vi "Finish.vi"(8 "error in (no error)":errorcluster, 11 "Turret in":refnum<class "Turret.lvclass">) -> (0 "error out":errorcluster, 3 "Turret out":refnum<class "Turret.lvclass">)   [LabVIEW 2019, in "Turret.lvlib" / "Turret.lvclass"]
uses:
  Turret.lvclass
  Turret.lvclass/Turret.ctl
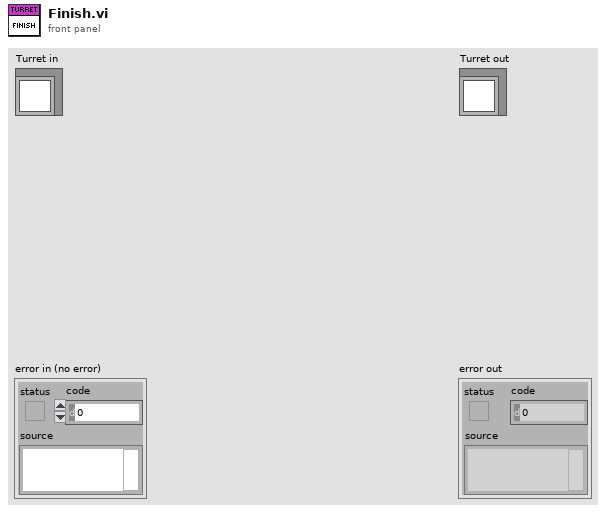
[diagram p1: front panel]
types:
  T1 = typedef "WPI_PotentiometerDevRef.ctl" = cluster{"DevStatus":errorcluster, "Analog Channel":T2, "Invert Output":bool}
  T2 = typedef "FPGA_AIChannel.ctl" = enum8{"AI 0", "AI 1", "AI 2", "AI 3", "AI MXP 0", "AI MXP 1", "AI MXP 2", "AI MXP 3", "Invalid"}
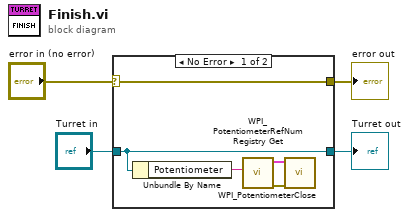
[diagram p0: block diagram]
diagram:
  n1 = case shown="No Error" "error in (no error)" {
    selector: "error in (no error)" -> [w9 w11]
    tunnel: [w9 w11] -> w3
    tunnel: [w6 w10] -> w1
    tunnel: "Turret in" -> [w6 w10]
    frame No Error {
      n2 = Unbundle By Name(w6) -> ("Potentiometer"=w5:string)
      n3 = call <vilib>:"WPI_PotentiometerRefNum Registry Get.vi"("refnum name"=w5) -> ("error out"=w8:errorcluster, "PotDevRef"=w7:T1)  [unwired: 9 in]
      n4 = call <vilib>:"WPI_PotentiometerClose.vi"("error in"=w8, "PotDevRef"=w7) -> ()  [unwired: 9 in, 1 out]
    }
    frame Error {
    }
  }
  "error out" <- w3
  "Turret out" <- w1
